vi "输入数据解析.vi"(0 "单个参数补充":dbl, 1 "从板号":dbl=1.0, 2 "主板二维码":string="BNET01", 3 "从板二维码":string="BNET01", 5 "主板引用":refnum<vi>, 7 "从板引用":refnum<vi>, 9 "主板选项":string="三级故障阀值", 11 "枚举":enum16{"主板", "从板"}(ring), 12 "快换":bool caption="快换写入") -> (4 "输出数组":dbl[][](array[numeric]), 6 "数组长度":dbl[](array[numeric]), 8 "循环次数":i32, 10 "命令":u32, 14 "名称":string[](array[string]), 15 "命令序号":u32[](array[numeric]))   [LabVIEW 2013] (continued)
                  frame "4", "铅酸" {
                  }
                  frame "5", "镍氢" {
                  }
                  frame "6", "钴酸锂" {
                  }
                  frame "7", "聚合物锂离子" {
                  }
                  frame "8", "钛酸锂" {
                  }
                  frame "9", "其他电池" {
                  }
                  frame "1", "磷酸铁锂", Default {
                  }
                }
                n5417 = Match Pattern(string=w14167, regular expression=w14166) -> (before substring=w14165:string, after substring=w14164:string)  [unwired: 3 out]
                n5418 = call "输入分辨率计算-EV05.vi"("1字节?"=FALSE, "数值"=w14204, "分辨率"=0.1) -> ("低字节"=w14175:dbl, "高字节1"=w14176:dbl)  [unwired: 2 in, 5 out]
                n5419 = Quotient & Remainder(x=w14183, y=w14198) -> (x-y*floor(x/y)=w14197:dbl, floor(x/y)=w14201:dbl)
                n5420 = Fract/Exp String To Number(string=w14168) -> (number=w14159:dbl)  [unwired: 4 out]
                n5421 = Quotient & Remainder(x=w14182, y=w14193) -> (x-y*floor(x/y)=w14189:dbl, floor(x/y)=w14190:dbl)
                n5422 = Quotient & Remainder(x=w14201, y=w14198) -> (x-y*floor(x/y)=w14196:dbl, floor(x/y)=w14200:dbl)
                n5423 = Fract/Exp String To Number(string=w14165) -> (number=w14158:dbl)  [unwired: 4 out]
                n5424 = Quotient & Remainder(x=w14190, y=w14193) -> (x-y*floor(x/y)=w14188:dbl, floor(x/y)=w14191:dbl)
                n5425 = call <vilib>:"Trim Whitespace.vi"("string"=w14164) -> ("trimmed string"=w14163:string)  [unwired: 1 in]
                n5426 = Quotient & Remainder(x=w14200, y=w14198) -> (x-y*floor(x/y)=w14195:dbl, floor(x/y)=w14199:dbl)
                n5427 = Quotient & Remainder(x=w14191, y=w14193) -> (x-y*floor(x/y)=w14187:dbl, floor(x/y)=w14192:dbl)
                n5428 = Quotient & Remainder(x=w14222, y=256.0) -> (x-y*floor(x/y)=w14224:dbl, floor(x/y)=w14225:dbl)
                n5429 = Fract/Exp String To Number(string=w14163) -> (number=w14157:dbl)  [unwired: 4 out]
                n5430 = Quotient & Remainder(x=w14199, y=w14198) -> (x-y*floor(x/y)=w14194:dbl)  [unwired: 1 out]
                n5431 = Quotient & Remainder(x=w14192, y=w14193) -> (x-y*floor(x/y)=w14186:dbl)  [unwired: 1 out]
                n5432 = Build Array(w14177, w14178, w14194, w14195, w14196, w14197, w14186, w14187, w14188, w14189, w14176, w14175, w14174, w14174, w14174, w14162, w14161, w14160, w14159, w14158, w14157) -> (w14173:dbl[])
                n5433 = Build Array(w14225, w14224, w14221, w14219, w14217) -> (w14223:dbl[])
                n5434 = Insert Into Array(array=w14223, new element=w14173) -> (w14206:dbl[])  [unwired: 1 in]
              }
              frame 1 {
                w14251 = 256.0 ("y")
                n5435 = Unbundle By Name(w14241) -> ("电池包组号"=w14252:string)
                n5436 = Decimal String To Number(string=w14252, default (0L)=0.0) -> (number=w14247:dbl)  [unwired: 1 in, 1 out]
                n5437 = Quotient & Remainder(x=w14247, y=w14251) -> (x-y*floor(x/y)=w14242:dbl, floor(x/y)=w14248:dbl)
                n5438 = Quotient & Remainder(x=w14248, y=w14251) -> (x-y*floor(x/y)=w14243:dbl, floor(x/y)=w14249:dbl)
                n5439 = Quotient & Remainder(x=w14249, y=w14251) -> (x-y*floor(x/y)=w14244:dbl, floor(x/y)=w14250:dbl)
                n5440 = Quotient & Remainder(x=w14250, y=w14251) -> (x-y*floor(x/y)=w14245:dbl)  [unwired: 1 out]
                n5441 = Build Array(w14245, w14244, w14243, w14242) -> (w14240:dbl[])
              }
              frame 2 {
                w14271 = 256.0 ("y")
                w14276 = 256.0 ("y")
                n5442 = Unbundle By Name(w14263) -> ("累计充电总安时"=w14260:dbl, "累计放电总安时"=w14259:dbl)
                n5443 = call "输入分辨率计算-EV05.vi"("1字节?"=TRUE, "数值 2"=w14259, "数值"=w14260, "分辨率"=0.001) -> ("高字节 2"=w14257:dbl, "高字节1"=w14258:dbl)  [unwired: 1 in, 5 out]
                n5444 = Quotient & Remainder(x=w14258, y=w14276) -> (x-y*floor(x/y)=w14275:dbl, floor(x/y)=w14279:dbl)
                n5445 = Quotient & Remainder(x=w14257, y=w14271) -> (x-y*floor(x/y)=w14267:dbl, floor(x/y)=w14268:dbl)
                n5446 = Quotient & Remainder(x=w14279, y=w14276) -> (x-y*floor(x/y)=w14274:dbl, floor(x/y)=w14278:dbl)
                n5447 = Quotient & Remainder(x=w14268, y=w14271) -> (x-y*floor(x/y)=w14266:dbl, floor(x/y)=w14269:dbl)
                n5448 = Quotient & Remainder(x=w14278, y=w14276) -> (x-y*floor(x/y)=w14273:dbl, floor(x/y)=w14277:dbl)
                n5449 = Quotient & Remainder(x=w14269, y=w14271) -> (x-y*floor(x/y)=w14265:dbl, floor(x/y)=w14270:dbl)
                n5450 = Quotient & Remainder(x=w14277, y=w14276) -> (x-y*floor(x/y)=w14272:dbl)  [unwired: 1 out]
                n5451 = Quotient & Remainder(x=w14270, y=w14271) -> (x-y*floor(x/y)=w14264:dbl)  [unwired: 1 out]
                n5452 = Build Array(w14272, w14273, w14274, w14275, w14264, w14265, w14266, w14267) -> (w14280:dbl[])
              }
              frame 3 {
                w14292 = 256.0 ("y")
                n5453 = Unbundle By Name(w14287) -> ("电池放空次数"=w14286:dbl, "电池充满次数"=w14285:dbl, "电池充电次数"=w14284:dbl)
                n5454 = Quotient & Remainder(x=w14286, y=w14292) -> (x-y*floor(x/y)=w14294:dbl, floor(x/y)=w14295:dbl)
                n5455 = Quotient & Remainder(x=w14285, y=w14292) -> (x-y*floor(x/y)=w14290:dbl, floor(x/y)=w14291:dbl)
                n5456 = Quotient & Remainder(x=w14284, y=w14292) -> (x-y*floor(x/y)=w14288:dbl, floor(x/y)=w14289:dbl)
                n5457 = Build Array(w14295, w14294, w14291, w14290, w14289, w14288) -> (w14293:dbl[])
              }
            }
          }
        }
        frame "电池包组号" {
          n5458 = Unbundle By Name(w14301) -> ("电池信息"=w14302:refnum<vi>)
          n5459 = property class="Clust (严格)"(reference=w14302) -> ("Value"=w14300:T7)  [unwired: 1 in, 2 out]
          n5460 = for {
            N: 1 -> [_]
            tunnel: [w14312] -> w14306 mode=indexing
            tunnel: [w14311] -> w14305 mode=indexing
            tunnel: [w14309] -> w14303 mode=indexing
            tunnel: w14300 -> [w14308]
            i -> [w14310]
            n5461 = case shown="0, 默认" w14310 {
              tunnel: [4 ("单个参数补充") 30 ("单个参数补充") 8 ("单个参数补充") 6 ("单个参数补充")] -> w14312
              tunnel: [2 ("命令序号") 1 ("命令序号") 4 ("命令序号") 5 ("命令序号")] -> w14311
              tunnel: [w14325 w14330 w14418 w14430] -> w14309
              tunnel: w14308 -> [w14324 w14339 w14401 w14424]
              frame 0, Default {
                w14322 = 256.0 ("y")
                n5462 = Unbundle By Name(w14324) -> ("电池包组号"=w14323:string)
                n5463 = Decimal String To Number(string=w14323, default (0L)=0.0) -> (number=w14318:dbl)  [unwired: 1 in, 1 out]
                n5464 = Quotient & Remainder(x=w14318, y=w14322) -> (x-y*floor(x/y)=w14313:dbl, floor(x/y)=w14319:dbl)
                n5465 = Quotient & Remainder(x=w14319, y=w14322) -> (x-y*floor(x/y)=w14314:dbl, floor(x/y)=w14320:dbl)
                n5466 = Quotient & Remainder(x=w14320, y=w14322) -> (x-y*floor(x/y)=w14315:dbl, floor(x/y)=w14321:dbl)
                n5467 = Quotient & Remainder(x=w14321, y=w14322) -> (x-y*floor(x/y)=w14316:dbl)  [unwired: 1 out]
                n5468 = Build Array(w14316, w14315, w14314, w14313) -> (w14325:dbl[])
              }
              frame 1 {
                w14352 = 2 ("偏移量(0)")
                w14349 = "-" ("正则表达式")
                n5469 = Unbundle By Name(w14339) -> ("电池包额定容量"=w14346:dbl, "电池包额定能量"=w14345:dbl, "电池包额定总电压"=w14340:dbl, "实际容量"=w14328:dbl)
                n5470 = Unbundle By Name(w14339) -> ("电池串联"=w14360:dbl, "电池并联"=w14359:dbl, "电池厂家"=w14358:string, "电池类型"=w14356:string, "电池生产日期"=w14354:string)
                n5471 = Match Pattern(string=w14354, regular expression=w14349) -> (before substring=w14353:string, after substring=w14350:string)  [unwired: 3 out]
                n5472 = Match Pattern(string=w14350, regular expression=w14349) -> (before substring=w14348:string, after substring=w14347:string)  [unwired: 3 out]
                n5473 = String Subset(string=w14353, offset (0)=w14352, length (rest)=w14352) -> (substring=w14351:string)
                n5474 = case shown="\"2\", \"盟固利\"" w14358 {
                  tunnel: [2 1] -> w14357
                  frame "2", "盟固利" {
                  }
                  frame "1", "普莱德", Default {
                  }
                }
                n5475 = case shown="\"9\", \"其他电池\"" w14356 {
                  tunnel: [2 3 4 5 6 7 8 9 1] -> w14355
                  frame "2", "锰酸锂" {
                  }
                  frame "3", "三元材料" {
                  }
                  frame "4", "铅酸" {
                  }
                  frame "5", "镍氢" {
                  }
                  frame "6", "钴酸锂" {
                  }
                  frame "7", "聚合物锂离子" {
                  }
                  frame "8", "钛酸锂" {
                  }
                  frame "9", "其他电池" {
                  }
                  frame "1", "磷酸铁锂", Default {
                  }
                }
                n5476 = call "输入分辨率计算-EV05.vi"("1字节?"=FALSE, "数值 2"=w14345, "数值"=w14346, "分辨率"=0.1) -> ("低字节 2"=w14335:dbl, "高字节 2"=w14336:dbl, "低字节"=w14337:dbl, "高字节1"=w14338:dbl)  [unwired: 1 in, 3 out]
                n5477 = call "输入分辨率计算-EV05.vi"("1字节?"=FALSE, "数值 2"=w14328, "数值"=w14340, "分辨率"=0.1) -> ("低字节 2"=w14331:dbl, "高字节 2"=w14332:dbl, "低字节"=w14333:dbl, "高字节1"=w14334:dbl)  [unwired: 1 in, 3 out]
                n5478 = Fract/Exp String To Number(string=w14351) -> (number=w14377:dbl)  [unwired: 1 in, 3 out]
                n5479 = Fract/Exp String To Number(string=w14348) -> (number=w14375:dbl)  [unwired: 4 out]
                n5480 = Fract/Exp String To Number(string=w14347) -> (number=w14373:dbl)  [unwired: 4 out]
                n5481 = Build Array(w14338, w14337, w14336, w14335, w14334, w14333, w14332, w14331) -> (w14329:dbl[])
                n5482 = Quotient & Remainder(x=w14360, y=256.0) -> (x-y*floor(x/y)=w14379:dbl, floor(x/y)=w14380:dbl)
                n5483 = call "二进制解析-8.6.vi"("索引"=7, "数值"=w14377) -> ("低位子数组"=w14368:i32[])  [unwired: 3 out]
                n5484 = call "二进制解析-8.6.vi"("索引"=4, "数值"=w14375) -> ("低位子数组"=w14371:i32[])  [unwired: 3 out]
                n5485 = call "二进制解析-8.6.vi"("索引"=5, "数值"=w14373) -> ("低位子数组"=w14365:i32[])  [unwired: 3 out]
                n5486 = Delete From Array(array=w14371, length=1 ("长度"), index=0 ("索引")) -> (deleted portion=w14367:i32[], array with subset deleted=w14366:i32[])
                n5487 = Insert Into Array(array=w14368, new element=w14367) -> (w14364:i32[])  [unwired: 1 in]
                n5488 = Insert Into Array(array=w14366, new element=w14365) -> (w14363:i32[])  [unwired: 1 in]
                n5489 = call "数值二进制转十进制-8.6.vi"("子数组"=w14364) -> ("十进制数值"=w14362:i32)  [unwired: 4 out]
                n5490 = call "数值二进制转十进制-8.6.vi"("子数组"=w14363) -> ("十进制数值"=w14361:i32)  [unwired: 4 out]
                n5491 = Build Array(w14380, w14379, w14359, w14357, w14355, w14362, w14361) -> (w14378:dbl[])
                n5492 = Insert Into Array(array=w14378, new element=w14329) -> (w14330:dbl[])  [unwired: 1 in]
              }
              frame 3 {
                w14409 = 256.0 ("y")
                w14414 = 256.0 ("y")
                n5493 = Unbundle By Name(w14401) -> ("累计充电总安时"=w14398:dbl, "累计放电总安时"=w14397:dbl)
                n5494 = call "输入分辨率计算-EV05.vi"("1字节?"=TRUE, "数值 2"=w14397, "数值"=w14398, "分辨率"=0.001) -> ("高字节 2"=w14395:dbl, "高字节1"=w14396:dbl)  [unwired: 1 in, 5 out]
                n5495 = Quotient & Remainder(x=w14396, y=w14414) -> (x-y*floor(x/y)=w14413:dbl, floor(x/y)=w14417:dbl)
                n5496 = Quotient & Remainder(x=w14395, y=w14409) -> (x-y*floor(x/y)=w14405:dbl, floor(x/y)=w14406:dbl)
                n5497 = Quotient & Remainder(x=w14417, y=w14414) -> (x-y*floor(x/y)=w14412:dbl, floor(x/y)=w14416:dbl)
                n5498 = Quotient & Remainder(x=w14406, y=w14409) -> (x-y*floor(x/y)=w14404:dbl, floor(x/y)=w14407:dbl)
                n5499 = Quotient & Remainder(x=w14416, y=w14414) -> (x-y*floor(x/y)=w14411:dbl, floor(x/y)=w14415:dbl)
                n5500 = Quotient & Remainder(x=w14407, y=w14409) -> (x-y*floor(x/y)=w14403:dbl, floor(x/y)=w14408:dbl)
                n5501 = Quotient & Remainder(x=w14415, y=w14414) -> (x-y*floor(x/y)=w14410:dbl)  [unwired: 1 out]
                n5502 = Quotient & Remainder(x=w14408, y=w14409) -> (x-y*floor(x/y)=w14402:dbl)  [unwired: 1 out]
                n5503 = Build Array(w14410, w14411, w14412, w14413, w14402, w14403, w14404, w14405) -> (w14418:dbl[])
              }
              frame 4 {
                w14429 = 256.0 ("y")
                n5504 = Unbundle By Name(w14424) -> ("电池放空次数"=w14423:dbl, "电池充满次数"=w14422:dbl, "电池充电次数"=w14421:dbl)
                n5505 = Quotient & Remainder(x=w14423, y=w14429) -> (x-y*floor(x/y)=w14431:dbl, floor(x/y)=w14432:dbl)
                n5506 = Quotient & Remainder(x=w14422, y=w14429) -> (x-y*floor(x/y)=w14427:dbl, floor(x/y)=w14428:dbl)
                n5507 = Quotient & Remainder(x=w14421, y=w14429) -> (x-y*floor(x/y)=w14425:dbl, floor(x/y)=w14426:dbl)
                n5508 = Build Array(w14432, w14431, w14428, w14427, w14426, w14425) -> (w14430:dbl[])
              }
            }
          }
        }
        frame "充放电安时" {
          n5509 = Unbundle By Name(w14438) -> ("电池信息"=w14439:refnum<vi>)
          n5510 = property class="Clust (严格)"(reference=w14439) -> ("Value"=w14437:T7)  [unwired: 1 in, 2 out]
          n5511 = for {
            N: 1 -> [_]
            tunnel: [w14449] -> w14443 mode=indexing
            tunnel: [w14448] -> w14442 mode=indexing
            tunnel: [w14446] -> w14440 mode=indexing
            tunnel: w14437 -> [w14445]
            i -> [w14447]
            n5512 = case shown="0, 默认" w14447 {
              tunnel: [8 ("单个参数补充") 30 ("单个参数补充") 4 ("单个参数补充") 6 ("单个参数补充")] -> w14449
              tunnel: [3 ("命令序号") 1 ("命令序号") 2 ("命令序号") 5 ("命令序号")] -> w14448
              tunnel: [w14473 w14478 w14555 w14567] -> w14446
              tunnel: w14445 -> [w14456 w14487 w14554 w14561]
              frame 0, Default {
                w14464 = 256.0 ("y")
                w14469 = 256.0 ("y")
                n5513 = Unbundle By Name(w14456) -> ("累计充电总安时"=w14453:dbl, "累计放电总安时"=w14452:dbl)
                n5514 = call "输入分辨率计算-EV05.vi"("1字节?"=TRUE, "数值 2"=w14452, "数值"=w14453, "分辨率"=0.001) -> ("高字节 2"=w14450:dbl, "高字节1"=w14451:dbl)  [unwired: 1 in, 5 out]
                n5515 = Quotient & Remainder(x=w14451, y=w14469) -> (x-y*floor(x/y)=w14468:dbl, floor(x/y)=w14472:dbl)
                n5516 = Quotient & Remainder(x=w14450, y=w14464) -> (x-y*floor(x/y)=w14460:dbl, floor(x/y)=w14461:dbl)
                n5517 = Quotient & Remainder(x=w14472, y=w14469) -> (x-y*floor(x/y)=w14467:dbl, floor(x/y)=w14471:dbl)
                n5518 = Quotient & Remainder(x=w14461, y=w14464) -> (x-y*floor(x/y)=w14459:dbl, floor(x/y)=w14462:dbl)
                n5519 = Quotient & Remainder(x=w14471, y=w14469) -> (x-y*floor(x/y)=w14466:dbl, floor(x/y)=w14470:dbl)
                n5520 = Quotient & Remainder(x=w14462, y=w14464) -> (x-y*floor(x/y)=w14458:dbl, floor(x/y)=w14463:dbl)
                n5521 = Quotient & Remainder(x=w14470, y=w14469) -> (x-y*floor(x/y)=w14465:dbl)  [unwired: 1 out]
                n5522 = Quotient & Remainder(x=w14463, y=w14464) -> (x-y*floor(x/y)=w14457:dbl)  [unwired: 1 out]
                n5523 = Build Array(w14465, w14466, w14467, w14468, w14457, w14458, w14459, w14460) -> (w14473:dbl[])
              }
              frame 1 {
                w14500 = 2 ("偏移量(0)")
                w14497 = "-" ("正则表达式")
                n5524 = Unbundle By Name(w14487) -> ("电池包额定容量"=w14494:dbl, "电池包额定能量"=w14493:dbl, "电池包额定总电压"=w14488:dbl, "实际容量"=w14476:dbl)
                n5525 = Unbundle By Name(w14487) -> ("电池串联"=w14508:dbl, "电池并联"=w14507:dbl, "电池厂家"=w14506:string, "电池类型"=w14504:string, "电池生产日期"=w14502:string)
                n5526 = Match Pattern(string=w14502, regular expression=w14497) -> (before substring=w14501:string, after substring=w14498:string)  [unwired: 3 out]
                n5527 = Match Pattern(string=w14498, regular expression=w14497) -> (before substring=w14496:string, after substring=w14495:string)  [unwired: 3 out]
                n5528 = String Subset(string=w14501, offset (0)=w14500, length (rest)=w14500) -> (substring=w14499:string)
                n5529 = case shown="\"2\", \"盟固利\"" w14506 {
                  tunnel: [2 1] -> w14505
                  frame "2", "盟固利" {
                  }
                  frame "1", "普莱德", Default {
                  }
                }
                n5530 = case shown="\"9\", \"其他电池\"" w14504 {
                  tunnel: [2 3 4 5 6 7 8 9 1] -> w14503
                  frame "2", "锰酸锂" {
                  }
                  frame "3", "三元材料" {
                  }
                  frame "4", "铅酸" {
                  }
                  frame "5", "镍氢" {
                  }
                  frame "6", "钴酸锂" {
                  }
                  frame "7", "聚合物锂离子" {
                  }
                  frame "8", "钛酸锂" {
                  }
                  frame "9", "其他电池" {
                  }
                  frame "1", "磷酸铁锂", Default {
                  }
                }
                n5531 = call "输入分辨率计算-EV05.vi"("1字节?"=FALSE, "数值 2"=w14493, "数值"=w14494, "分辨率"=0.1) -> ("低字节 2"=w14483:dbl, "高字节 2"=w14484:dbl, "低字节"=w14485:dbl, "高字节1"=w14486:dbl)  [unwired: 1 in, 3 out]
                n5532 = call "输入分辨率计算-EV05.vi"("1字节?"=FALSE, "数值 2"=w14476, "数值"=w14488, "分辨率"=0.1) -> ("低字节 2"=w14479:dbl, "高字节 2"=w14480:dbl, "低字节"=w14481:dbl, "高字节1"=w14482:dbl)  [unwired: 1 in, 3 out]
                n5533 = Fract/Exp String To Number(string=w14499) -> (number=w14525:dbl)  [unwired: 1 in, 3 out]
                n5534 = Fract/Exp String To Number(string=w14496) -> (number=w14523:dbl)  [unwired: 4 out]
                n5535 = Fract/Exp String To Number(string=w14495) -> (number=w14521:dbl)  [unwired: 4 out]
                n5536 = Build Array(w14486, w14485, w14484, w14483, w14482, w14481, w14480, w14479) -> (w14477:dbl[])
                n5537 = Quotient & Remainder(x=w14508, y=256.0) -> (x-y*floor(x/y)=w14527:dbl, floor(x/y)=w14528:dbl)
                n5538 = call "二进制解析-8.6.vi"("索引"=7, "数值"=w14525) -> ("低位子数组"=w14516:i32[])  [unwired: 3 out]
                n5539 = call "二进制解析-8.6.vi"("索引"=4, "数值"=w14523) -> ("低位子数组"=w14519:i32[])  [unwired: 3 out]
                n5540 = call "二进制解析-8.6.vi"("索引"=5, "数值"=w14521) -> ("低位子数组"=w14513:i32[])  [unwired: 3 out]
                n5541 = Delete From Array(array=w14519, length=1 ("长度"), index=0 ("索引")) -> (deleted portion=w14515:i32[], array with subset deleted=w14514:i32[])
                n5542 = Insert Into Array(array=w14516, new element=w14515) -> (w14512:i32[])  [unwired: 1 in]
                n5543 = Insert Into Array(array=w14514, new element=w14513) -> (w14511:i32[])  [unwired: 1 in]
                n5544 = call "数值二进制转十进制-8.6.vi"("子数组"=w14512) -> ("十进制数值"=w14510:i32)  [unwired: 4 out]
                n5545 = call "数值二进制转十进制-8.6.vi"("子数组"=w14511) -> ("十进制数值"=w14509:i32)  [unwired: 4 out]
                n5546 = Build Array(w14528, w14527, w14507, w14505, w14503, w14510, w14509) -> (w14526:dbl[])
                n5547 = Insert Into Array(array=w14526, new element=w14477) -> (w14478:dbl[])  [unwired: 1 in]
              }
              frame 3 {
                w14548 = 256.0 ("y")
                n5548 = Unbundle By Name(w14554) -> ("电池包组号"=w14553:string)
                n5549 = Match Pattern(string=w14553, regular expression="-" ("正则表达式")) -> (before substring=w14551:string, after substring=w14550:string)  [unwired: 3 out]
                n5550 = Fract/Exp String To Number(string=w14551) -> (number=w14549:dbl)  [unwired: 1 in, 3 out]
                n5551 = Fract/Exp String To Number(string=w14550) -> (number=w14547:dbl)  [unwired: 4 out]
                n5552 = Quotient & Remainder(x=w14547, y=w14548) -> (x-y*floor(x/y)=w14545:dbl, floor(x/y)=w14546:dbl)
                n5553 = Quotient & Remainder(x=w14549, y=w14548) -> (x-y*floor(x/y)=w14543:dbl, floor(x/y)=w14544:dbl)
                n5554 = Build Array(w14546, w14545, w14544, w14543) -> (w14555:dbl[])
              }
              frame 4 {
                w14566 = 256.0 ("y")
                n5555 = Unbundle By Name(w14561) -> ("电池放空次数"=w14560:dbl, "电池充满次数"=w14559:dbl, "电池充电次数"=w14558:dbl)
                n5556 = Quotient & Remainder(x=w14560, y=w14566) -> (x-y*floor(x/y)=w14568:dbl, floor(x/y)=w14569:dbl)
                n5557 = Quotient & Remainder(x=w14559, y=w14566) -> (x-y*floor(x/y)=w14564:dbl, floor(x/y)=w14565:dbl)
                n5558 = Quotient & Remainder(x=w14558, y=w14566) -> (x-y*floor(x/y)=w14562:dbl, floor(x/y)=w14563:dbl)
                n5559 = Build Array(w14569, w14568, w14565, w14564, w14563, w14562) -> (w14567:dbl[])
              }
            }
          }
        }
        frame "电池充放电次数" {
          n5560 = Unbundle By Name(w14575) -> ("电池信息"=w14576:refnum<vi>)
          n5561 = property class="Clust (严格)"(reference=w14576) -> ("Value"=w14574:T7)  [unwired: 1 in, 2 out]
          n5562 = for {
            N: 1 -> [_]
            tunnel: [w14586] -> w14580 mode=indexing
            tunnel: [w14585] -> w14579 mode=indexing
            tunnel: [w14583] -> w14577 mode=indexing
            tunnel: w14574 -> [w14582]
            i -> [w14584]
            n5563 = case shown="0, 默认" w14584 {
              tunnel: [6 ("单个参数补充") 30 ("单个参数补充") 4 ("单个参数补充") 8 ("单个参数补充")] -> w14586
              tunnel: [4 ("命令序号") 1 ("命令序号") 2 ("命令序号") 3 ("命令序号")] -> w14585
              tunnel: [w14596 w14603 w14680 w14706] -> w14583
              tunnel: w14582 -> [w14590 w14612 w14679 w14689]
              frame 0, Default {
                w14595 = 256.0 ("y")
                n5564 = Unbundle By Name(w14590) -> ("电池放空次数"=w14589:dbl, "电池充满次数"=w14588:dbl, "电池充电次数"=w14587:dbl)
                n5565 = Quotient & Remainder(x=w14589, y=w14595) -> (x-y*floor(x/y)=w14597:dbl, floor(x/y)=w14598:dbl)
                n5566 = Quotient & Remainder(x=w14588, y=w14595) -> (x-y*floor(x/y)=w14593:dbl, floor(x/y)=w14594:dbl)
                n5567 = Quotient & Remainder(x=w14587, y=w14595) -> (x-y*floor(x/y)=w14591:dbl, floor(x/y)=w14592:dbl)
                n5568 = Build Array(w14598, w14597, w14594, w14593, w14592, w14591) -> (w14596:dbl[])
              }
              frame 1 {
                w14625 = 2 ("偏移量(0)")
                w14622 = "-" ("正则表达式")
                n5569 = Unbundle By Name(w14612) -> ("电池包额定容量"=w14619:dbl, "电池包额定能量"=w14618:dbl, "电池包额定总电压"=w14613:dbl, "实际容量"=w14601:dbl)
                n5570 = Unbundle By Name(w14612) -> ("电池串联"=w14633:dbl, "电池并联"=w14632:dbl, "电池厂家"=w14631:string, "电池类型"=w14629:string, "电池生产日期"=w14627:string)
                n5571 = Match Pattern(string=w14627, regular expression=w14622) -> (before substring=w14626:string, after substring=w14623:string)  [unwired: 3 out]
                n5572 = Match Pattern(string=w14623, regular expression=w14622) -> (before substring=w14621:string, after substring=w14620:string)  [unwired: 3 out]
                n5573 = String Subset(string=w14626, offset (0)=w14625, length (rest)=w14625) -> (substring=w14624:string)
                n5574 = case shown="\"2\", \"盟固利\"" w14631 {
                  tunnel: [2 1] -> w14630
                  frame "2", "盟固利" {
                  }
                  frame "1", "普莱德", Default {
                  }
                }
                n5575 = case shown="\"9\", \"其他电池\"" w14629 {
                  tunnel: [2 3 4 5 6 7 8 9 1] -> w14628
                  frame "2", "锰酸锂" {
                  }
                  frame "3", "三元材料" {
                  }
                  frame "4", "铅酸" {
                  }
                  frame "5", "镍氢" {
                  }
                  frame "6", "钴酸锂" {
                  }
                  frame "7", "聚合物锂离子" {
                  }
                  frame "8", "钛酸锂" {
                  }
                  frame "9", "其他电池" {
                  }
                  frame "1", "磷酸铁锂", Default {
                  }
                }
                n5576 = call "输入分辨率计算-EV05.vi"("1字节?"=FALSE, "数值 2"=w14618, "数值"=w14619, "分辨率"=0.1) -> ("低字节 2"=w14608:dbl, "高字节 2"=w14609:dbl, "低字节"=w14610:dbl, "高字节1"=w14611:dbl)  [unwired: 1 in, 3 out]
                n5577 = call "输入分辨率计算-EV05.vi"("1字节?"=FALSE, "数值 2"=w14601, "数值"=w14613, "分辨率"=0.1) -> ("低字节 2"=w14604:dbl, "高字节 2"=w14605:dbl, "低字节"=w14606:dbl, "高字节1"=w14607:dbl)  [unwired: 1 in, 3 out]
                n5578 = Fract/Exp String To Number(string=w14624) -> (number=w14650:dbl)  [unwired: 1 in, 3 out]
                n5579 = Fract/Exp String To Number(string=w14621) -> (number=w14648:dbl)  [unwired: 4 out]
                n5580 = Fract/Exp String To Number(string=w14620) -> (number=w14646:dbl)  [unwired: 4 out]
                n5581 = Build Array(w14611, w14610, w14609, w14608, w14607, w14606, w14605, w14604) -> (w14602:dbl[])
                n5582 = Quotient & Remainder(x=w14633, y=256.0) -> (x-y*floor(x/y)=w14652:dbl, floor(x/y)=w14653:dbl)
                n5583 = call "二进制解析-8.6.vi"("索引"=7, "数值"=w14650) -> ("低位子数组"=w14641:i32[])  [unwired: 3 out]
                n5584 = call "二进制解析-8.6.vi"("索引"=4, "数值"=w14648) -> ("低位子数组"=w14644:i32[])  [unwired: 3 out]
                n5585 = call "二进制解析-8.6.vi"("索引"=5, "数值"=w14646) -> ("低位子数组"=w14638:i32[])  [unwired: 3 out]
                n5586 = Delete From Array(array=w14644, length=1 ("长度"), index=0 ("索引")) -> (deleted portion=w14640:i32[], array with subset deleted=w14639:i32[])
                n5587 = Insert Into Array(array=w14641, new element=w14640) -> (w14637:i32[])  [unwired: 1 in]
                n5588 = Insert Into Array(array=w14639, new element=w14638) -> (w14636:i32[])  [unwired: 1 in]
                n5589 = call "数值二进制转十进制-8.6.vi"("子数组"=w14637) -> ("十进制数值"=w14635:i32)  [unwired: 4 out]
                n5590 = call "数值二进制转十进制-8.6.vi"("子数组"=w14636) -> ("十进制数值"=w14634:i32)  [unwired: 4 out]
                n5591 = Build Array(w14653, w14652, w14632, w14630, w14628, w14635, w14634) -> (w14651:dbl[])
                n5592 = Insert Into Array(array=w14651, new element=w14602) -> (w14603:dbl[])  [unwired: 1 in]
              }
              frame 3 {
                w14673 = 256.0 ("y")
                n5593 = Unbundle By Name(w14679) -> ("电池包组号"=w14678:string)
                n5594 = Match Pattern(string=w14678, regular expression="-" ("正则表达式")) -> (before substring=w14676:string, after substring=w14675:string)  [unwired: 3 out]
                n5595 = Fract/Exp String To Number(string=w14676) -> (number=w14674:dbl)  [unwired: 1 in, 3 out]
                n5596 = Fract/Exp String To Number(string=w14675) -> (number=w14672:dbl)  [unwired: 4 out]
                n5597 = Quotient & Remainder(x=w14672, y=w14673) -> (x-y*floor(x/y)=w14670:dbl, floor(x/y)=w14671:dbl)
                n5598 = Quotient & Remainder(x=w14674, y=w14673) -> (x-y*floor(x/y)=w14668:dbl, floor(x/y)=w14669:dbl)
                n5599 = Build Array(w14671, w14670, w14669, w14668) -> (w14680:dbl[])
              }
              frame 4 {
                w14697 = 256.0 ("y")
                w14702 = 256.0 ("y")
                n5600 = Unbundle By Name(w14689) -> ("累计充电总安时"=w14686:dbl, "累计放电总安时"=w14685:dbl)
                n5601 = call "输入分辨率计算-EV05.vi"("1字节?"=TRUE, "数值 2"=w14685, "数值"=w14686, "分辨率"=0.001) -> ("高字节 2"=w14683:dbl, "高字节1"=w14684:dbl)  [unwired: 1 in, 5 out]
                n5602 = Quotient & Remainder(x=w14684, y=w14702) -> (x-y*floor(x/y)=w14701:dbl, floor(x/y)=w14705:dbl)
                n5603 = Quotient & Remainder(x=w14683, y=w14697) -> (x-y*floor(x/y)=w14693:dbl, floor(x/y)=w14694:dbl)
                n5604 = Quotient & Remainder(x=w14705, y=w14702) -> (x-y*floor(x/y)=w14700:dbl, floor(x/y)=w14704:dbl)
                n5605 = Quotient & Remainder(x=w14694, y=w14697) -> (x-y*floor(x/y)=w14692:dbl, floor(x/y)=w14695:dbl)
                n5606 = Quotient & Remainder(x=w14704, y=w14702) -> (x-y*floor(x/y)=w14699:dbl, floor(x/y)=w14703:dbl)
                n5607 = Quotient & Remainder(x=w14695, y=w14697) -> (x-y*floor(x/y)=w14691:dbl, floor(x/y)=w14696:dbl)
                n5608 = Quotient & Remainder(x=w14703, y=w14702) -> (x-y*floor(x/y)=w14698:dbl)  [unwired: 1 out]
                n5609 = Quotient & Remainder(x=w14696, y=w14697) -> (x-y*floor(x/y)=w14690:dbl)  [unwired: 1 out]
                n5610 = Build Array(w14698, w14699, w14700, w14701, w14690, w14691, w14692, w14693) -> (w14706:dbl[])
              }
            }
          }
        }
        frame "历史信息" {
          n5611 = disable-structure shown="禁用" {
            disable-tunnel: [u32 163 ("命令序号") _] -> w14713
            disable-tunnel: [w14718 _] -> w14712
            disable-tunnel: [w14717 _] -> w14711
            disable-tunnel: w14710 -> [w14716 _]
            disable-tunnel: [w14714 _] -> w14709
            frame Disabled {
              n5612 = for {
                N: 4 -> [_]
                tunnel: [w14724] -> w14718 mode=indexing
                tunnel: [w14723] -> w14717 mode=indexing
                tunnel: w14716 -> [w14721]
                tunnel: [w14720] -> w14714 mode=indexing
                i -> [w14722]
                n5613 = case shown="0, 默认" w14722 {
                  tunnel: [14 ("单个参数补充") 9 ("单个参数补充") 12 ("单个参数补充") 12 ("单个参数补充")] -> w14724
                  tunnel: [1 ("命令序号") 2 ("命令序号") 3 ("命令序号") 4 ("命令序号")] -> w14723
                  tunnel: w14721 -> [w14732 w14767 w14798 w14826]
                  tunnel: [w14726 w14761 w14792 w14824] -> w14720
                  frame 0, Default {
                    n5614 = Index Array(array=w14732, index (col)=22 ("禁用的索引 (列)")) -> (element=w14731)  [unwired: 1 in]
                    n5615 = Array Subset(array=w14731, index=0 ("索引"), length=7 ("长度")) -> (w14728:void[])
                    n5616 = Fract/Exp String To Number(string=w14728) -> (number=w14727:dbl[])  [unwired: 1 in, 3 out]
                    n5617 = for {
                      tunnel: w14727 -> [w14744] mode=indexing
                      shift-right: [w14739] -> w14726
                      shift-left: dbl[] [] -> [w14738]
                      i -> [w14745]
                      n5618 = case shown="6" w14745 {
                        tunnel: [0.001 ("分辨率") 0.001 ("分辨率") 1.0 ("分辨率") 0.001 ("分辨率") 0.001 ("分辨率") 0.1 ("分辨率") 0.1 ("分辨率")] -> w14737
                        tunnel: [0.0 ("分辨率") 0.0 ("分辨率") 0.0 ("分辨率") 0.0 ("分辨率") 0.0 ("分辨率") 0.0 ("分辨率") 0.0 ("分辨率")] -> w14736
                        frame 0, Default {
                        }
                        frame 1 {
                        }
                        frame 2 {
                        }
                        frame 3 {
                        }
                        frame 4 {
                        }
                        frame 5 {
                        }
                        frame 6 {
                        }
                      }
                      n5619 = call "输入分辨率计算-EV05.vi"("1字节?"=FALSE, "数值"=w14744, "偏移量"=w14736, "分辨率"=w14737) -> ("低字节"=w14741:dbl, "高字节1"=w14742:dbl)  [unwired: 1 in, 5 out]
                      n5620 = Build Array(w14742, w14741) -> (w14740:dbl[])
                      n5621 = Insert Into Array(array=w14738, new element=w14740) -> (w14739:dbl[])  [unwired: 1 in]
                    }
                  }
                  frame 1 {
                    n5622 = Index Array(array=w14767, index (col)=22 ("禁用的索引 (列)")) -> (element=w14766)  [unwired: 1 in]
                    n5623 = Array Subset(array=w14766, index=8 ("索引"), length=9 ("长度")) -> (w14763:void[])
                    n5624 = Fract/Exp String To Number(string=w14763) -> (number=w14762:dbl[])  [unwired: 1 in, 3 out]
                    n5625 = for {
                      tunnel: w14762 -> [w14777] mode=indexing
                      shift-right: [w14775] -> w14761
                      shift-left: dbl[] [] -> [w14774]
                      i -> [w14778]
                      n5626 = case shown="0, 默认" w14778 {
                        tunnel: [1.0 ("分辨率") 1.0 ("分辨率") 1.0 ("分辨率") 1.0 ("分辨率") 1.0 ("分辨率") 1.0 ("分辨率")] -> w14773
                        tunnel: [-40.0 ("分辨率") -40.0 ("分辨率") 0.0 ("分辨率") -40.0 ("分辨率") -40.0 ("分辨率") 0.0 ("分辨率")] -> w14772
                        frame 0, Default {
                        }
                        frame 1 {
                        }
                        frame 2 {
                        }
                        frame 3 {
                        }
                        frame 4 {
                        }
                        frame 5..8 {
                        }
                      }
                      n5627 = call "输入分辨率计算-EV05.vi"("1字节?"=TRUE, "数值"=w14777, "偏移量"=w14772, "分辨率"=w14773) -> ("高字节1"=w14771:dbl)  [unwired: 1 in, 6 out]
                      n5628 = Insert Into Array(array=w14774, new element=w14771) -> (w14775:dbl[])  [unwired: 1 in]
                    }
                  }
                  frame 2 {
                    n5629 = Index Array(array=w14798, index (col)=22 ("禁用的索引 (列)")) -> (element=w14797)  [unwired: 1 in]
                    n5630 = Array Subset(array=w14797, index=17 ("索引"), length=6 ("长度")) -> (w14794:void[])
                    n5631 = Fract/Exp String To Number(string=w14794) -> (number=w14793:dbl[])  [unwired: 1 in, 3 out]
                    n5632 = for {
                      tunnel: w14793 -> [w14810] mode=indexing
                      shift-right: [w14805] -> w14792
                      shift-left: dbl[] [] -> [w14804]
                      i -> [w14811]
                      n5633 = case shown="4, 5" w14811 {
                        tunnel: [0.01 ("分辨率") 0.01 ("分辨率") 0.1 ("分辨率") 0.1 ("分辨率") 1.0 ("分辨率")] -> w14803
                        tunnel: [-300.0 ("分辨率") -300.0 ("分辨率") -3000.0 ("分辨率") -3000.0 ("分辨率") 0.0 ("分辨率")] -> w14802
                        frame 0, Default {
                        }
                        frame 1 {
                        }
                        frame 2 {
                        }
                        frame 3 {
                        }
                        frame 4, 5 {
                        }
                      }
                      n5634 = call "输入分辨率计算-EV05.vi"("1字节?"=FALSE, "数值"=w14810, "偏移量"=w14802, "分辨率"=w14803) -> ("低字节"=w14807:dbl, "高字节1"=w14808:dbl)  [unwired: 1 in, 5 out]
                      n5635 = Build Array(w14808, w14807) -> (w14806:dbl[])
                      n5636 = Insert Into Array(array=w14804, new element=w14806) -> (w14805:dbl[])  [unwired: 1 in]
                    }
                  }
                  frame 3 {
                    w14832 = 256.0 ("y")
                    w14844 = 256.0 ("y")
                    w14849 = 256.0 ("y")
                    n5637 = Index Array(array=w14826, index (col)=22 ("禁用的索引 (列)")) -> (element=w14859)  [unwired: 1 in]
                    n5638 = Index Array(array=w14859, index #1=23 ("索引"), index #2=24 ("索引"), index #3=25 ("索引")) -> (element #1=w14825, element #2=w14854, element #3=w14853)
                    n5639 = Fract/Exp String To Number(string=w14854) -> (number=w14840:dbl)  [unwired: 1 in, 3 out]
                    n5640 = Fract/Exp String To Number(string=w14825) -> (number=w14855:dbl)  [unwired: 1 in, 3 out]
                    n5641 = Fract/Exp String To Number(string=w14853) -> (number=w14831:dbl)  [unwired: 4 out]
                    n5642 = Quotient & Remainder(x=w14855, y=w14849) -> (x-y*floor(x/y)=w14848:dbl, floor(x/y)=w14852:dbl)
                    n5643 = Quotient & Remainder(x=w14840, y=w14844) -> (x-y*floor(x/y)=w14839:dbl, floor(x/y)=w14841:dbl)
                    n5644 = Quotient & Remainder(x=w14831, y=w14832) -> (x-y*floor(x/y)=w14830:dbl, floor(x/y)=w14835:dbl)
                    n5645 = Quotient & Remainder(x=w14852, y=w14849) -> (x-y*floor(x/y)=w14847:dbl, floor(x/y)=w14851:dbl)
                    n5646 = Quotient & Remainder(x=w14841, y=w14844) -> (x-y*floor(x/y)=w14838:dbl, floor(x/y)=w14842:dbl)
                    n5647 = Quotient & Remainder(x=w14835, y=w14832) -> (x-y*floor(x/y)=w14829:dbl, floor(x/y)=w14834:dbl)
                    n5648 = Quotient & Remainder(x=w14851, y=w14849) -> (x-y*floor(x/y)=w14846:dbl, floor(x/y)=w14850:dbl)
                    n5649 = Quotient & Remainder(x=w14842, y=w14844) -> (x-y*floor(x/y)=w14837:dbl, floor(x/y)=w14843:dbl)
                    n5650 = Quotient & Remainder(x=w14834, y=w14832) -> (x-y*floor(x/y)=w14828:dbl, floor(x/y)=w14833:dbl)
                    n5651 = Quotient & Remainder(x=w14850, y=w14849) -> (x-y*floor(x/y)=w14845:dbl)  [unwired: 1 out]
                    n5652 = Quotient & Remainder(x=w14843, y=w14844) -> (x-y*floor(x/y)=w14836:dbl)  [unwired: 1 out]
                    n5653 = Quotient & Remainder(x=w14833, y=w14832) -> (x-y*floor(x/y)=w14827:dbl)  [unwired: 1 out]
                    n5654 = Build Array(w14845, w14846, w14847, w14848, w14836, w14837, w14838, w14839, w14827, w14828, w14829, w14830) -> (w14824:dbl[])
                  }
                }
              }
            }
            frame Enabled {
            }
          }
        }
      }
    }
    frame "从板" {
      n5655 = property class="Clust (严格)"(reference="从板引用") -> ("Value"=w14863:T1)  [unwired: 1 in, 2 out]
      n5656 = case shown="\"从板信息\"" w14872 {
        tunnel: w14863 -> [_ w14882 w14892 w14929 w15065 w15093 w15131 w15167 w15347 w15522 w15697 w15872 w16047 w16222 w16397 w16575 w16641 w16743 w16845 w16947 w17049 w17151 w17253 w17355 w17457 w17559 w17661 w17763 w17865 w17967 w18069 w18171 w18273 w18375 w18477 w18567 w18657 w18747 w18812 w18878 w19079 w19178 w19277 w19375 w19575 w19718 w19861 w20004 w20147 _ w20305]
        tunnel: [_ w14879 w14895 w14932 w15068 w15096 w15134 w15170 w15350 w15525 w15700 w15875 w16050 w16225 w16400 w16577 w16643 w16745 w16847 w16949 w17051 w17153 w17255 w17357 w17459 w17561 w17663 w17765 w17867 w17969 w18071 w18173 w18275 w18377 w18479 w18569 w18659 w18749 w18814 w18877 w19078 w19177 w19276 w19374 w19574 w19717 w19860 w20003 w20146 w20290 w20304] -> w14871
        tunnel: [_ u32 32 ("命令序号") u32 32 ("命令序号") u32 32 ("命令序号") u32 32 ("命令序号") u32 32 ("命令序号") u32 32 ("命令序号") u32 32 ("命令序号") u32 32 ("命令序号") u32 32 ("命令序号") u32 32 ("命令序号") u32 32 ("命令序号") u32 32 ("命令序号") u32 32 ("命令序号") u32 32 ("命令序号") u32 34 ("命令序号") u32 34 ("命令序号") u32 34 ("命令序号") u32 34 ("命令序号") u32 34 ("命令序号") u32 34 ("命令序号") u32 34 ("命令序号") u32 34 ("命令序号") u32 34 ("命令序号") u32 34 ("命令序号") u32 34 ("命令序号") u32 34 ("命令序号") u32 34 ("命令序号") u32 34 ("命令序号") u32 34 ("命令序号") u32 34 ("命令序号") u32 34 ("命令序号") u32 34 ("命令序号") u32 34 ("命令序号") u32 34 ("命令序号") u32 34 ("命令序号") u32 34 ("命令序号") u32 34 ("命令序号") u32 34 ("命令序号") w18875 u32 38 ("命令序号") u32 38 ("命令序号") u32 38 ("命令序号") w19372 w19572 w19715 w19858 w20001 w20144 u32 42 ("命令序号") w20302] -> w14870
        tunnel: [_ u32[] [6] w14893 w14930 w15066 w15094 w15132 w15168 w15348 w15523 w15698 w15873 w16048 w16223 w16398 u32[] [1] u32[] [1] u32[] [2] u32[] [3] u32[] [1] u32[] [2] u32[] [3] u32[] [1] u32[] [2] u32[] [3] u32[] [1] u32[] [2] u32[] [3] u32[] [1] u32[] [2] u32[] [3] u32[] [1] u32[] [2] u32[] [3] u32[] [1] u32[] [2] u32[] [3] u32[] [2] u32[] [3] w18879 w19080 w19179 w19278 w19376 w19576 w19719 w19862 w20005 w20148 w20287 w20306] -> w14869
        tunnel: [_ dbl[] [1.0] w14894 w14931 w15067 w15095 w15133 w15169 w15349 w15524 w15699 w15874 w16049 w16224 w16399 dbl[] [15.0] dbl[] [15.0] dbl[] [15.0] dbl[] [15.0] dbl[] [15.0] dbl[] [15.0] dbl[] [15.0] dbl[] [15.0] dbl[] [15.0] dbl[] [15.0] dbl[] [15.0] dbl[] [15.0] dbl[] [15.0] dbl[] [15.0] dbl[] [15.0] dbl[] [15.0] dbl[] [15.0] dbl[] [15.0] dbl[] [15.0] dbl[] [15.0] dbl[] [15.0] dbl[] [15.0] dbl[] [15.0] dbl[] [15.0] w18880 w19081 w19180 w19279 w19377 w19577 w19720 w19863 w20006 w20149 w20288 w20307] -> w14868
        tunnel: w14867 -> [_ _ _ _ _ _ _ w15171 w15351 w15526 w15701 w15876 w16051 w16226 w16401 _ _ _ _ _ _ _ _ _ _ _ _ _ _ _ _ _ _ _ _ _ _ _ _ _ _ _ _ _ _ _ _ _ _ _ _]
        tunnel: w14866 -> [_ _ _ _ _ _ _ _ _ _ _ _ _ _ _ _ _ _ _ _ _ _ _ _ _ _ _ _ _ _ _ _ _ _ _ _ _ _ _ w18876 _ _ _ w19373 w19573 w19716 w19859 w20002 w20145 _ w20303]
        tunnel: w14865 -> [_ w14875 _ w14927 _ _ _ _ _ _ _ _ _ _ _ _ _ _ _ _ _ _ _ _ _ _ _ _ _ _ _ _ _ _ _ _ _ _ _ _ _ _ _ _ _ _ _ _ _ _ _]
        tunnel: [_ 1 1 5 1 1 1 1 1 1 1 1 1 1 1 1 1 1 1 1 1 1 1 1 1 1 1 1 1 1 1 1 1 1 1 1 1 1 1 w18874 w19076 w19175 w19274 w19371 1 1 1 1 1 1 1] -> w14862
        tunnel: [_ string[] ["从板号"] string[] ["电压起始值"] w14926 string[] ["通道电压节数"] string[] ["保险位置"] string[] ["温度起始值"] string[] ["加热控制参数"] string[] ["加热控制参数"] string[] ["加热控制参数"] string[] ["加热控制参数"] string[] ["加热控制参数"] string[] ["加热控制参数"] string[] ["加热控制参数"] string[] ["加热控制参数"] string[] ["一级故障阀值"] string[] ["一级故障阀值"] string[] ["二级故障阀值"] string[] ["三级故障阀值"] string[] ["一级故障阀值"] string[] ["二级故障阀值"] string[] ["三级故障阀值"] string[] ["一级故障阀值"] string[] ["二级故障阀值"] string[] ["三级故障阀值"] string[] ["一级故障阀值"] string[] ["二级故障阀值"] string[] ["三级故障阀值"] string[] ["一级故障阀值"] string[] ["二级故障阀值"] string[] ["三级故障阀值"] string[] ["一级故障阀值"] string[] ["二级故障阀值"] string[] ["三级故障阀值"] string[] ["一级故障阀值"] string[] ["二级故障阀值"] string[] ["三级故障阀值"] string[] ["二级故障阀值"] string[] ["三级故障阀值"] w18873 w19075 w19174 w19273 w19370 string[] ["电池包序号"] string[] ["充放电安时"] string[] ["充电次数时间"] string[] ["SOC"] string[] ["车牌号"] w20289 string[] ["充电参数"]] -> w14861
        frame "假", Default {
        }
        frame "从板号" {
          n5657 = disable-structure shown="启用" {
            disable-tunnel: w14882 -> [w14888 _]
            disable-tunnel: [w14883 w14889] -> w14881
            disable-tunnel: w14875 -> [_ w14889]
            frame Disabled {
              n5658 = Index Array(array=w14888, index (col)=4 ("禁用的索引 (列)")) -> (element=w14886)  [unwired: 1 in]
              n5659 = Index Array(array=w14886, index=1 ("索引")) -> (element=w14884)
              n5660 = Fract/Exp String To Number(string=w14884) -> (number=w14883:dbl)  [unwired: 4 out]
            }
            frame Enabled {
            }
          }
          n5661 = Build Array(w14881) -> (w14880:dbl[])
          n5662 = Build Array(w14880) -> (w14879:dbl[][])
        }
        frame "电压个数" {
          n5663 = for {
            N: 1 -> [_]
            tunnel: [w14901] -> w14895 mode=indexing
            tunnel: [w14900] -> w14894 mode=indexing
            tunnel: [w14899] -> w14893 mode=indexing
            tunnel: w14892 -> [w14898]
            i -> [w14902]
            n5664 = case shown="0, 默认" w14902 {
              tunnel: w14898 -> [w14910]
              tunnel: [w14905] -> w14901
              tunnel: [4.0 ("y")] -> w14900
              tunnel: [u32 1 ("命令序号")] -> w14899
              frame 0, Default {
                n5665 = Unbundle By Name(w14910) -> ("项目信息 2"=w14911:refnum<vi>)
                n5666 = property class="Tbl (严格)"(reference=w14911) -> ("Value"=w14909:string[][])  [unwired: 1 in, 2 out]
                n5667 = Index Array(array=w14909, index (col)=1 ("禁用的索引 (列)")) -> (element=w14913:string[])  [unwired: 1 in]
                n5668 = Array Subset(array=w14913, index=0 ("索引"), length=2.0 ("y")) -> (w14914:string[])
                n5669 = Fract/Exp String To Number(string=w14914) -> (number=w14907:dbl[])  [unwired: 4 out]
                n5670 = for {
                  N: 1 -> [_]
                  tunnel: w14907 -> [w14925] mode=indexing
                  shift-right: [w14920] -> w14905
                  shift-left: dbl[] [] -> [w14919]
                  n5671 = Quotient & Remainder(x=w14925, y=256.0) -> (x-y*floor(x/y)=w14922:dbl, floor(x/y)=w14923:dbl)
                  n5672 = Build Array(w14923, w14922, 0.0 ("元素"), 1.0 ("元素")) -> (w14921:dbl[])
                  n5673 = Insert Into Array(array=w14919, new element=w14921) -> (w14920:dbl[])  [unwired: 1 in]
                }
              }
            }
          }
        }
        frame "从板信息" {
          n5674 = for {
            N: 6 -> [_]
            tunnel: [w14940] -> w14932 mode=indexing
            tunnel: [w14939] -> w14931 mode=indexing
            tunnel: [w14938] -> w14930 mode=indexing
            tunnel: w14929 -> [w14937]
            tunnel: w14927 -> [w14936]
            tunnel: [w14935] -> w14926 mode=indexing
            i -> [w14941]
            n5675 = case shown="5" w14941 {
              tunnel: w14937 -> [w14950 w14972 w14990 w15016 w15043 _]
              tunnel: [w14945 w14967 w14984 w15014 w15042 w15059] -> w14940
              tunnel: [4.0 ("y") 20.0 ("y") 10.0 ("y") 4.0 ("y") 7.0 ("y") 1.0 ("y")] -> w14939
              tunnel: [u32 1 ("命令序号") u32 2 ("命令序号") u32 3 ("命令序号") u32 4 ("命令序号") u32 5 ("命令序号") u32 6 ("命令序号")] -> w14938
              tunnel: w14936 -> [_ _ _ _ _ w15062]
              tunnel: ["电压起始值" "通道电压节数" "保险位置" "温度起始值" "加热控制参数" "从板号"] -> w14935
              frame 1, Default {
                # "起始位置改为1"
                n5676 = Unbundle By Name(w14950) -> ("项目信息 2"=w14951:refnum<vi>)
                n5677 = property class="Tbl (严格)"(reference=w14951) -> ("Value"=w14949:string[][])  [unwired: 1 in, 2 out]
                n5678 = Index Array(array=w14949, index (col)=1 ("禁用的索引 (列)")) -> (element=w14953:string[])  [unwired: 1 in]
                n5679 = Array Subset(array=w14953, index=0 ("索引"), length=1.0 ("y")) -> (w14954:string[])
                n5680 = Fract/Exp String To Number(string=w14954) -> (number=w14947:dbl[])  [unwired: 4 out]
                n5681 = for {
                  N: 1 -> [_]
                  tunnel: w14947 -> [w14965] mode=indexing
                  shift-right: [w14960] -> w14945
                  shift-left: dbl[] [] -> [w14959]
                  n5682 = Quotient & Remainder(x=w14965, y=256.0) -> (x-y*floor(x/y)=w14962:dbl, floor(x/y)=w14963:dbl)
                  n5683 = Build Array(w14963, w14962, 0.0 ("元素"), 1.0 ("元素")) -> (w14961:dbl[])
                  n5684 = Insert Into Array(array=w14959, new element=w14961) -> (w14960:dbl[])  [unwired: 1 in]
                }
              }
              frame 2 {
                n5685 = Unbundle By Name(w14972) -> ("项目信息 2"=w14975:refnum<vi>)
                n5686 = property class="Tbl (严格)"(reference=w14975) -> ("Value"=w14974:string[][])  [unwired: 1 in, 2 out]
                n5687 = Index Array(array=w14974, index (col)=1 ("禁用的索引 (列)")) -> (element=w14976:string[])  [unwired: 1 in]
                n5688 = Array Subset(array=w14976, index=22 ("索引"), length=5.0 ("y")) -> (w14977:string[])
                n5689 = Fract/Exp String To Number(string=w14977) -> (number=w14968:dbl[])  [unwired: 4 out]
                n5690 = for {
                  N: 20 -> [_]
                  tunnel: w14968 -> [w14981] mode=indexing
                  tunnel: [w14980] -> w14967 mode=indexing
                  w14982 = 12.0 ("y")
                  n5691 = Greater?(x=w14981, y=w14982) -> (0:w14983:bool)
                  n5692 = Select(t=w14982, s=w14983, f=w14981) -> (s? t:f=w14980:dbl)
                }
              }
              frame 3 {
                n5693 = Unbundle By Name(w14990) -> ("项目信息 2"=w14993:refnum<vi>)
                n5694 = property class="Tbl (严格)"(reference=w14993) -> ("Value"=w14992:string[][])  [unwired: 1 in, 2 out]
                n5695 = Index Array(array=w14992, index (col)=1 ("禁用的索引 (列)")) -> (element=w14994:string[])  [unwired: 1 in]
                n5696 = Array Subset(array=w14994, index=2 ("索引"), length=20.0 ("y")) -> (w14995:string[])
                n5697 = Fract/Exp String To Number(string=w14995) -> (number=w14986:dbl[])  [unwired: 4 out]
                n5698 = for {
                  N: 10 -> [_]
                  tunnel: w14986 -> [w15007]
                  tunnel: [w14998] -> w14984 mode=indexing
                  i -> [w15009]
                  w15002 = 4 ("索引")
                  n5699 = Multiply(x=w15009, y=2) -> (x*y=w15006:i32)
                  n5700 = Increment(x=w15006) -> (x+1=w15005:i32)
                  n5701 = Index Array(array=w15007, index #1=w15006, index #2=w15005) -> (element #1=w15004:dbl, element #2=w15003:dbl)
                  n5702 = call "二进制解析-8.6.vi"("索引"=w15002, "数值"=w15004) -> ("低位子数组"=w15001:i32[])  [unwired: 1 in, 2 out]
                  n5703 = call "二进制解析-8.6.vi"("索引"=w15002, "数值"=w15003) -> ("低位子数组"=w15000:i32[])  [unwired: 1 in, 2 out]
                  n5704 = Insert Into Array(array=w15001, new element=w15000) -> (w14999:i32[])  [unwired: 1 in]
                  n5705 = call "数值二进制转十进制-8.6.vi"("子数组"=w14999) -> ("十进制数值"=w14998:i32)  [unwired: 4 in]
                }
              }
              frame 4 {
                n5706 = Unbundle By Name(w15016) -> ("项目信息 2"=w15020:refnum<vi>)
                n5707 = property class="Tbl (严格)"(reference=w15020) -> ("Value"=w15019:string[][])  [unwired: 1 in, 2 out]
                n5708 = Index Array(array=w15019, index (col)=1 ("禁用的索引 (列)")) -> (element=w15021:string[])  [unwired: 1 in]
                n5709 = Array Subset(array=w15021, index=1 ("索引"), length=1.0 ("y")) -> (w15022:string[])
                n5710 = Fract/Exp String To Number(string=w15022) -> (number=w15018:dbl[])  [unwired: 4 out]
                n5711 = for {
                  N: 1 -> [_]
                  tunnel: w15018 -> [w15033] mode=indexing
                  shift-right: [w15028] -> w15014
                  shift-left: dbl[] [] -> [w15027]
                  n5712 = Quotient & Remainder(x=w15033, y=256.0) -> (x-y*floor(x/y)=w15030:dbl, floor(x/y)=w15031:dbl)
                  n5713 = Build Array(w15031, w15030, 0.0 ("元素"), 1.0 ("元素")) -> (w15029:dbl[])
                  n5714 = Insert Into Array(array=w15027, new element=w15029) -> (w15028:dbl[])  [unwired: 1 in]
                }
              }
              frame 5 {
                n5715 = Unbundle By Name(w15043) -> ("加热控制参数"=w15057:refnum<vi>)
                n5716 = property class="Clust (严格)"(reference=w15057) -> ("Value"=w15056:T5)  [unwired: 1 in, 2 out]
                n5717 = Unbundle(w15056) -> ("风机开启温度"=w15051:dbl, "风机关闭温度"=w15050:dbl, "加热开启温度"=w15047:dbl, "加热关闭温度"=w15046:dbl, "风机开启温差"=w15038:dbl, "风机关闭温差"=w15036:dbl, "加热关闭温差"=w15034:dbl)
                n5718 = call "输入分辨率计算-EV05.vi"("1字节?"=TRUE, "数值 2"=w15046, "数值"=w15047, "偏移量"=-40.0, "分辨率"=1.0) -> ("高字节 2"=w15035:dbl, "高字节1"=w15037:dbl)  [unwired: 5 out]
                n5719 = call "输入分辨率计算-EV05.vi"("1字节?"=TRUE, "数值 2"=w15050, "数值"=w15051, "偏移量"=-40.0, "分辨率"=1.0) -> ("高字节 2"=w15045:dbl, "高字节1"=w15044:dbl)  [unwired: 5 out]
                n5720 = Build Array(w15044, w15045, w15038, w15036, w15037, w15035, w15034) -> (w15042:dbl[])
              }
              frame 0 {
                n5721 = Build Array(w15062) -> (w15059:dbl[])
              }
            }
          }
        }
        frame "通道电压节数" {
          n5722 = for {
            N: 1 -> [_]
            tunnel: [w15074] -> w15068 mode=indexing
            tunnel: [w15073] -> w15067 mode=indexing
            tunnel: [w15072] -> w15066 mode=indexing
            tunnel: w15065 -> [w15071]
            i -> [w15075]
            n5723 = case shown="0, 默认" w15075 {
              tunnel: w15071 -> [w15080]
              tunnel: [w15076] -> w15074
              tunnel: [w15078] -> w15073
              tunnel: [2 ("命令序号")] -> w15072
              frame 0, Default {
                w15078 = 20.0 ("y")
                n5724 = Unbundle By Name(w15080) -> ("项目信息 2"=w15081:refnum<vi>)
                n5725 = property class="Tbl (严格)"(reference=w15081) -> ("Value"=w15079:string[][])  [unwired: 1 in, 2 out]
                n5726 = Index Array(array=w15079, index (col)=1 ("禁用的索引 (列)")) -> (element=w15083:string[])  [unwired: 1 in]
                n5727 = Array Subset(array=w15083, index=22 ("索引"), length=w15078) -> (w15084:string[])
                n5728 = Fract/Exp String To Number(string=w15084) -> (number=w15077:dbl[])  [unwired: 4 out]
                n5729 = for {
                  tunnel: w15077 -> [w15088] mode=indexing
                  tunnel: [w15087] -> w15076 mode=indexing
                  w15089 = 12.0 ("y")
                  n5730 = Greater?(x=w15088, y=w15089) -> (0:w15090:bool)
                  n5731 = Select(t=w15089, s=w15090, f=w15088) -> (s? t:f=w15087:dbl)
                }
              }
            }
          }
        }
        frame "保险位置" {
          n5732 = for {
            N: 1 -> [_]
            tunnel: [w15102] -> w15096 mode=indexing
            tunnel: [w15101] -> w15095 mode=indexing
            tunnel: [w15100] -> w15094 mode=indexing
            tunnel: w15093 -> [w15099]
            i -> [w15103]
            n5733 = case shown="0, 默认" w15103 {
              tunnel: w15099 -> [w15110]
              tunnel: [w15104] -> w15102
              tunnel: [10.0 ("y")] -> w15101
